vi "Show View.vi"(8 "error in (no error)":errorcluster, 9 "Custom Position":cluster{"Top":i16, "Left":i16}, 10 "Position":T1, 11 "IViewable in":refnum<class "IViewable.lvclass">) -> (0 "error out":errorcluster, 3 "IViewable out":refnum<class "IViewable.lvclass">)   [LabVIEW 2015, in "IViewable.lvlib" / "IViewable.lvclass"]
uses:
  IViewable.lvclass
  View Position Enum.ctl
  IViewable.lvclass/IViewable.ctl
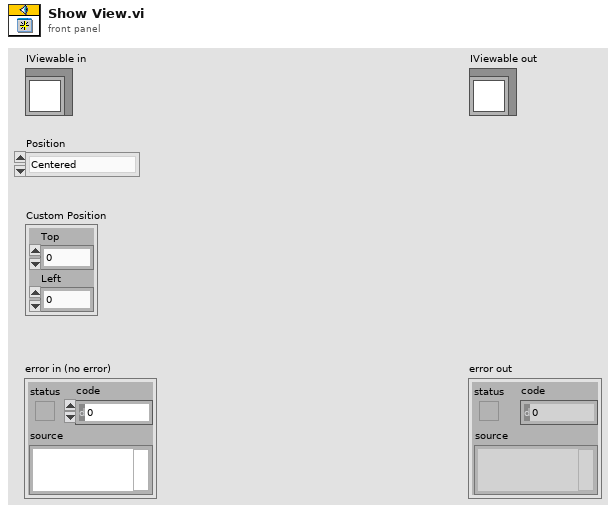
[diagram p1: front panel]
types:
  T1 = typedef "IViewable.lvlib/IViewable.lvclass/View Position Enum.ctl" = enum16{"Centered", "Maximized", "Minimized", "Custom", "Unchanged"}
  T2 = enum32{"Invalid", "Standard", "Closed", "Hidden", "Minimized", "Maximized"}
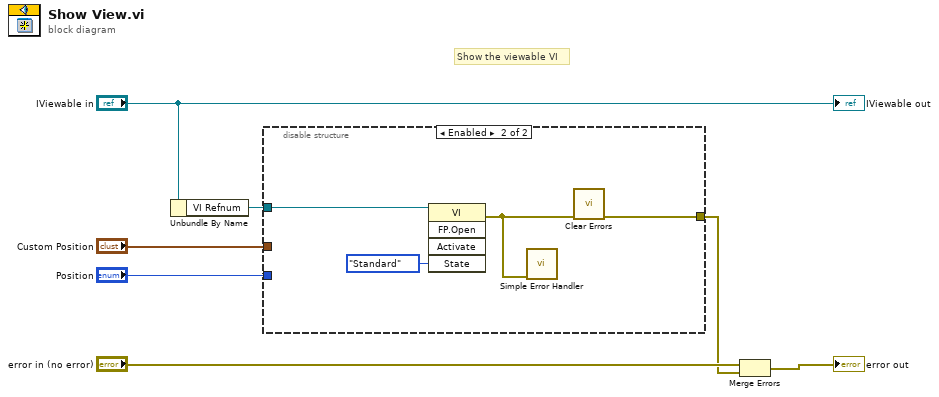
[diagram p0: block diagram]
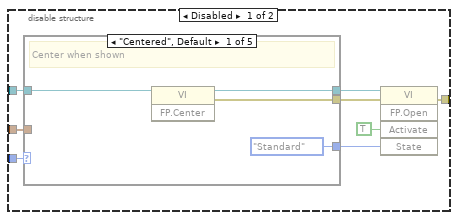
[diagram p2: hidden frame]
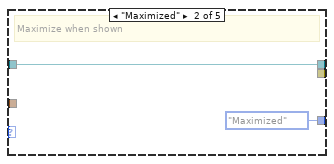
[diagram p3: hidden frame]
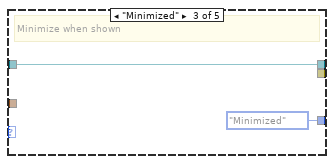
[diagram p4: hidden frame]
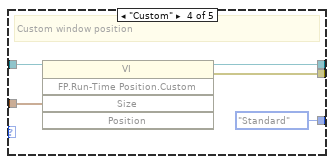
[diagram p5: hidden frame]
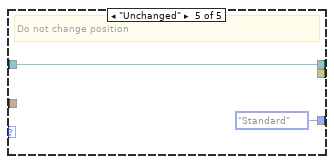
[diagram p6: hidden frame]
diagram:
  # "Show the viewable VI"
  n1 = Unbundle By Name("IViewable in") -> ("VI Refnum"=w4:refnum<vi>)
  n2 = disable-structure shown="Enabled" {
    disable-tunnel: w4 -> [w15 w34]
    disable-tunnel: [w14 w32] -> w3
    disable-tunnel: "Position" -> [w11 _]
    disable-tunnel: "Custom Position" -> [w10 _]
    frame Disabled {
      n3 = case shown="\"Centered\", Default" w11 {
        tunnel: w15 -> [w19 w21 w23 w28 w30]
        tunnel: [w18 w21 w23 w27 w30] -> w13
        tunnel: [w17 _ _ w26 _] -> w12
        tunnel: w10 -> [_ _ _ w25 _]
        tunnel: [T2."Standard" ("State") T2."Maximized" ("State") T2."Minimized" ("State") T2."Standard" ("State") T2."Standard" ("State")] -> w8
        frame "Centered", Default {
          # "Center when shown"
          n4 = invoke class="VI" method="FP.Center"(reference=w19) -> (reference out=w18:refnum<vi>, error out=w17:errorcluster)  [unwired: 2 in, 1 out]
        }
        frame "Maximized" {
          # "Maximize when shown"
        }
        frame "Minimized" {
          # "Minimize when shown"
        }
        frame "Custom" {
          # "Custom window position"
          n5 = invoke class="VI" method="FP.Run-Time Position.Custom"(reference=w28, "Size"=w25) -> (reference out=w27:refnum<vi>, error out=w26:errorcluster)  [unwired: 3 in, 3 out]
        }
        frame "Unchanged" {
          # "Do not change position"
        }
      }
      n6 = invoke class="VI" method="FP.Open"(reference=w13, error in=w12, "Activate"=TRUE ("Activate?"), "State"=w8) -> (error out=w14:errorcluster)  [unwired: 1 in, 4 out]
    }
    frame Enabled {
      n7 = invoke class="VI" method="FP.Open"(reference=w34, "State"=T2."Standard") -> (error out=w31:errorcluster)  [unwired: 3 in, 4 out]
      n8 = call <vilib>:"Simple Error Handler.vi"("error in (no error)"=w31) -> ()  [unwired: 4 in, 5 out]
      n9 = call <vilib>:"Clear Errors.vi"("error in (no error)"=w31) -> ("error out"=w32:errorcluster)  [unwired: 5 in, 1 out]
    }
  }
  n10 = Merge Errors("error in (no error)", w3) -> (→"error out":errorcluster)
  "IViewable out" <- "IViewable in"
